vi "Save code byte.vi"(8 "Last buffer element?":bool, 9 "Code":u8, 10 "Code index in":i32, 11 "Buffer in":u8[](array[numeric])) -> (2 "Code index out":i32, 3 "Buffer out":u8[](array[numeric]))   [LabVIEW 2020, in "COBS.lvlib"]
uses:
  COBS.lvlib
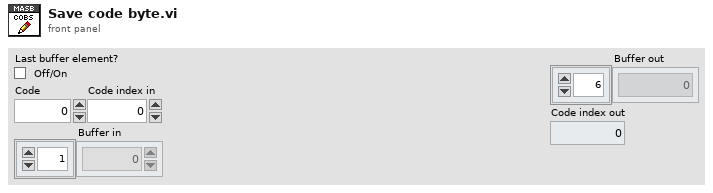
[diagram p1: front panel]
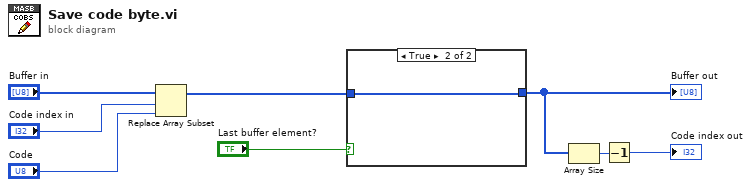
[diagram p0: block diagram]
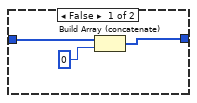
[diagram p2: hidden frame]
diagram:
  n1 = Replace Array Subset(array="Buffer in", new element="Code", index="Code index in") -> (w4:u8[])
  n2 = case shown="True" "Last buffer element?" {
    tunnel: w4 -> [w11 w12]
    tunnel: [w9 w12] -> w7
    frame False {
      n3 = Build Array (concatenate)(w11, u8 0) -> (w9:u8[])
    }
    frame True {
    }
  }
  "Buffer out" <- w7
  n4 = Array Size(array=w7) -> (size(s)=w5:i32)
  n5 = Decrement(x=w5) -> (x-1=→"Code index out":i32)
